vi "Recipe compare.vi"(8 "Recipe 2":T1={"SEM Scan Parameters"={"X size (um)"=20.0, "Y size (um)"=20.0, "X center (um)"=0.0, "Y center (um)"=0.0, "X size (V)"=6.190428211586902, "X size auto"=TRUE, "X stig"=[[0.0]], "Y stig"=[[0.0]], "X aln"=[[0.0]], "Y aln"=[[0.0]], "Scan rate (Hz)"=10000000, "Oversampling"=5, "Oversampling auto"=TRUE, "Frame line rampdown ratio"=0.1, "Pixel size (nm)"=10.0, "WD (mm)"=[[3.0]], "X tiles"=1, "Y tiles"=1, "Overlap (um)"=1.0, "Interlaced"=TRUE, "dX (um)"=0.0, "dY (um)"=0.0}, "Detector Information"={"Brightness A"=30.0, "Contrast A"=25.0, "Detector B name"="ESB", "Brightness B"=40.0, "Contrast B"=50.0, "Detector C name"="Detector C", "Detector D name"="Detector D"}, "SEM Options"={"GetInfo"=TRUE, "Set Det A para"=TRUE, "Set WD"=FALSE, "Set Mag"=TRUE, "Set stig"=FALSE, "Set aln"=FALSE, "Display"=TRUE, "Save"=TRUE, "Detector A"=TRUE, "Detector B"=FALSE, "Detector C"=FALSE, "Detector D"=FALSE, "Inverse A"=FALSE, "Inverse B"=FALSE, "Inverse C"=FALSE, "Inverse D"=FALSE, "Inverse PNG"=TRUE, "Freeze"=TRUE, "PNG only"=FALSE, "Upload"=TRUE, "Delete after upload"=FALSE}, "Keep aspect ratio"=TRUE, "Show Focus Index"=TRUE, "Focus Index primary grid center"=TRUE, "Focus Index grid X"=1, "Focus Index grid Y"=1, "Focus Index primary X grid"=0, "Focus Index primary Y grid"=0, "Image fit to"=0, "File Information"={"File path"=path "E:/Images", "Notes"="", "Save recipe"=FALSE, "Load recipe"=FALSE, "Sample ID"=""}, "Low mag SEM"={"Low mag scan"=TRUE, "Prior to main scan"=FALSE, "Low mag interval"=1, "Low mag scan FOV (micron)"=200.0, "Low mag scan rate (Hz)"=1000000, "Show HM box"=TRUE}, "Mid Mag SEM"={"Mid mag scan"=FALSE, "Prior to main scan"=FALSE, "Mid mag interval"=500, "X size (um)"=6144.0, "Y size (um)"=6144.0, "X center (um)"=0.0, "Y center (um)"=0.0, "Mid mag scan rate (Hz)"=1000000, "Pixel size (nm)"=10.0, "Show MM box"=TRUE}, "FIB-SEM Angle"=90.0, "Milling para"={"X resolution"=4096, "Y resolution"=100001, "X offset (um)"=0.0, "Y offset (um)"=0.0, "X center (um)"=0.0, "Y center (um)"=0.0, "X size (um)"=250.0, "Y size (um)"=250.0, "UL-Ang"=90.0, "UR-Ang"=90.0, "Line milling time (s)"=5.0, "Auto pause"=FALSE, "Lines auto pause"=1, "Mill from Bottom"=FALSE, "FIB FOV (um)"=500.0, "SEM on"=FALSE, "Mill start from Last"=FALSE, "FIB PID on"=FALSE, "FIB PID reset"=FALSE, "FIB PID measured"=0, "FIB PID target"=0.0, "FIB PID target slope"=0.0, "FIB PID P"=0.0, "FIB PID I"=0.0, "FIB PID D"=0.0}, "FI Detector"=0, "Auto Optimzation"=TRUE, "Images per Auto Optimization"=200, "AF Range (nm)"=1800.0, "AF Steps"=7, "AS Range (%)"=0.6, "AS Steps"=7, "AA Range (%)"=3.0, "AA Steps"=7, "X shift (nm/frame)"=0.0, "Y shift (nm/frame)"=0.0, "FIB Settings"={"Z-step (nm)"=2.5, "Enable alarm"=TRUE, "Label"="Emission Alarm (nA)", "Emission min"=1.2, "Emission max"=2.2, "Auto reheat"=FALSE}, "FIB Y zoom pixel (nm)"=20.0, "Mail server"="mail.hhmi.org", "Email Alert Recipents"=["xuc@janelia.hhmi.org"], "Alert Settings"={"3D imaging paused alarm"=TRUE, "FIB emission limit warning"=TRUE, "Low limit"=17.0, "High limit"=23.0, "Specimen current alarm "=TRUE, "Beam dump alarm"=TRUE, "EHT off alarm"=TRUE, "Temperature alarm"=TRUE, "Pause 3D-ING"=FALSE, "Low limit (F)"=70.0, "High limit (F)"=80.0, "Temp limit auto"=TRUE, "Delta (F)"=0.2, "Gradient limit (F/min)"=0.03, "SW error warning"=TRUE, "Focus index warning"=TRUE, "Focus index low limit"=0.1, "Focus index stop limit"=0.0, "Run Auto Stig"=FALSE, "FI low limit auto"=TRUE, "FI stop limit auto"=TRUE}, "Reheat Parameters"={"Filament I (A)"=3.0, "Reheat time (s)"=45.0, "Emission (uA)"=2.2, "Calculate V/I slope"=TRUE, "Pre-calc delay (min)"=5.0, "Disable Reheat Retries"=FALSE, "Restore Voltages"=TRUE}, "Start FIB HV DataLog"=FALSE, "Interval (s)"=60} {"SEM Scan Parameters"."dX (um)" step=1 format="%.2f"; "SEM Scan Parameters"."dY (um)" step=1 format="%.2f"; "SEM Scan Parameters"."WD (mm)" format="%.1f"; "SEM Scan Parameters"."Y aln" format="%.1f"; "SEM Scan Parameters"."X aln" format="%.1f"; "SEM Scan Parameters"."Y stig" format="%.1f"; "SEM Scan Parameters"."X stig" format="%.1f"; "SEM Scan Parameters"."Overlap (um)" min=0; "SEM Scan Parameters"."Y tiles" min=1; "SEM Scan Parameters"."X tiles" min=1; "SEM Scan Parameters"."X size (um)" format="%.2f"; "SEM Scan Parameters"."Y size (um)" format="%.2f"; "SEM Scan Parameters"."Frame line rampdown ratio" min=0 max=1 step=0.05 format="%.2g"; "SEM Scan Parameters"."X center (um)" step=1.0 format="%.2f"; "SEM Scan Parameters"."Y center (um)" step=1.0 format="%.2f"; "SEM Scan Parameters"."X size (V)" format="%_4g"; "SEM Scan Parameters"."Scan rate (Hz)" max=4000000 step=100000 format="%.2e"; "Reheat Parameters"."Pre-calc delay (min)" format="%.2f"; "Reheat Parameters"."Emission (uA)" format="%.1f"; "Reheat Parameters"."Filament I (A)" format="%.2f"; "Reheat Parameters"."Reheat time (s)" format="%.1f"; "Image fit to" items=["Width", "Height"]; "Mid Mag SEM"."X center (um)" step=1.0 format="%.4f"; "Mid Mag SEM"."Y center (um)" step=1.0 format="%.4f"; "Mid Mag SEM"."Mid mag interval" min=1 step=1; "Mid Mag SEM"."Mid mag scan rate (Hz)" max=4000000 step=100000 format="%.2e"; "Alert Settings"."Focus index stop limit" format="%_3g"; "Milling para"."FIB PID measured" items=["Spec.", "B.D."]; "Milling para"."UR-Ang" format="%.2f"; "Milling para"."UL-Ang" format="%.2f"; "Milling para"."Y offset (um)" step=0.02 format="%.3g"; "Milling para"."X offset (um)" step=1 format="%.3g"; "Milling para"."FIB FOV (um)" format="%.3g"; "Milling para"."Line milling time (s)" format="%.1f"; "Milling para"."Y center (um)" format="%#.3g"; "Milling para"."X center (um)" format="%#.3g"; "Focus Index grid X" min=1; "Focus Index grid Y" min=1; "FIB Y zoom pixel (nm)" format="%.1g"; "FIB Settings"."Emission min" format="%.1g"; "FIB Settings"."Emission max" format="%.1g"; "X shift (nm/frame)" step=0.1; "Y shift (nm/frame)" step=0.1; "FI Detector" items=["A", "B", "C", "D"]; "Low mag SEM"."Low mag interval" min=1 step=1; "Low mag SEM"."Low mag scan rate (Hz)" max=4000000 step=100000 format="%.2e"; "Low mag SEM"."Low mag scan FOV (micron)" step=50.0; "FIB-SEM Angle" min=0.0 max=90.0}, 11 "Recipe 1":T1={"SEM Scan Parameters"={"X size (um)"=20.0, "Y size (um)"=20.0, "X center (um)"=0.0, "Y center (um)"=0.0, "X size (V)"=6.190428211586902, "X size auto"=TRUE, "X stig"=[[0.0]], "Y stig"=[[0.0]], "X aln"=[[0.0]], "Y aln"=[[0.0]], "Scan rate (Hz)"=10000000, "Oversampling"=5, "Oversampling auto"=TRUE, "Frame line rampdown ratio"=0.1, "Pixel size (nm)"=10.0, "WD (mm)"=[[3.0]], "X tiles"=1, "Y tiles"=1, "Overlap (um)"=1.0, "Interlaced"=TRUE, "dX (um)"=0.0, "dY (um)"=0.0}, "Detector Information"={"Brightness A"=30.0, "Contrast A"=25.0, "Detector B name"="ESB", "Brightness B"=40.0, "Contrast B"=50.0, "Detector C name"="Detector C", "Detector D name"="Detector D"}, "SEM Options"={"GetInfo"=TRUE, "Set Det A para"=TRUE, "Set WD"=FALSE, "Set Mag"=TRUE, "Set stig"=FALSE, "Set aln"=FALSE, "Display"=TRUE, "Save"=TRUE, "Detector A"=TRUE, "Detector B"=FALSE, "Detector C"=FALSE, "Detector D"=FALSE, "Inverse A"=FALSE, "Inverse B"=FALSE, "Inverse C"=FALSE, "Inverse D"=FALSE, "Inverse PNG"=TRUE, "Freeze"=TRUE, "PNG only"=FALSE, "Upload"=TRUE, "Delete after upload"=FALSE}, "Keep aspect ratio"=TRUE, "Show Focus Index"=TRUE, "Focus Index primary grid center"=TRUE, "Focus Index grid X"=1, "Focus Index grid Y"=1, "Focus Index primary X grid"=0, "Focus Index primary Y grid"=0, "Image fit to"=0, "File Information"={"File path"=path "E:/Images", "Notes"="", "Save recipe"=FALSE, "Load recipe"=FALSE, "Sample ID"=""}, "Low mag SEM"={"Low mag scan"=TRUE, "Prior to main scan"=FALSE, "Low mag interval"=1, "Low mag scan FOV (micron)"=200.0, "Low mag scan rate (Hz)"=1000000, "Show HM box"=TRUE}, "Mid Mag SEM"={"Mid mag scan"=FALSE, "Prior to main scan"=FALSE, "Mid mag interval"=500, "X size (um)"=6144.0, "Y size (um)"=6144.0, "X center (um)"=0.0, "Y center (um)"=0.0, "Mid mag scan rate (Hz)"=1000000, "Pixel size (nm)"=10.0, "Show MM box"=TRUE}, "FIB-SEM Angle"=90.0, "Milling para"={"X resolution"=4096, "Y resolution"=100001, "X offset (um)"=0.0, "Y offset (um)"=0.0, "X center (um)"=0.0, "Y center (um)"=0.0, "X size (um)"=250.0, "Y size (um)"=250.0, "UL-Ang"=90.0, "UR-Ang"=90.0, "Line milling time (s)"=5.0, "Auto pause"=FALSE, "Lines auto pause"=1, "Mill from Bottom"=FALSE, "FIB FOV (um)"=500.0, "SEM on"=FALSE, "Mill start from Last"=FALSE, "FIB PID on"=FALSE, "FIB PID reset"=FALSE, "FIB PID measured"=0, "FIB PID target"=0.0, "FIB PID target slope"=0.0, "FIB PID P"=0.0, "FIB PID I"=0.0, "FIB PID D"=0.0}, "FI Detector"=0, "Auto Optimzation"=TRUE, "Images per Auto Optimization"=200, "AF Range (nm)"=1800.0, "AF Steps"=7, "AS Range (%)"=0.6, "AS Steps"=7, "AA Range (%)"=3.0, "AA Steps"=7, "X shift (nm/frame)"=0.0, "Y shift (nm/frame)"=0.0, "FIB Settings"={"Z-step (nm)"=2.5, "Enable alarm"=TRUE, "Label"="Emission Alarm (nA)", "Emission min"=1.2, "Emission max"=2.2, "Auto reheat"=FALSE}, "FIB Y zoom pixel (nm)"=20.0, "Mail server"="mail.hhmi.org", "Email Alert Recipents"=["xuc@janelia.hhmi.org"], "Alert Settings"={"3D imaging paused alarm"=TRUE, "FIB emission limit warning"=TRUE, "Low limit"=17.0, "High limit"=23.0, "Specimen current alarm "=TRUE, "Beam dump alarm"=TRUE, "EHT off alarm"=TRUE, "Temperature alarm"=TRUE, "Pause 3D-ING"=FALSE, "Low limit (F)"=70.0, "High limit (F)"=80.0, "Temp limit auto"=TRUE, "Delta (F)"=0.2, "Gradient limit (F/min)"=0.03, "SW error warning"=TRUE, "Focus index warning"=TRUE, "Focus index low limit"=0.1, "Focus index stop limit"=0.0, "Run Auto Stig"=FALSE, "FI low limit auto"=TRUE, "FI stop limit auto"=TRUE}, "Reheat Parameters"={"Filament I (A)"=3.0, "Reheat time (s)"=45.0, "Emission (uA)"=2.2, "Calculate V/I slope"=TRUE, "Pre-calc delay (min)"=5.0, "Disable Reheat Retries"=FALSE, "Restore Voltages"=TRUE}, "Start FIB HV DataLog"=FALSE, "Interval (s)"=60} {"SEM Scan Parameters"."dX (um)" step=1 format="%.2f"; "SEM Scan Parameters"."dY (um)" step=1 format="%.2f"; "SEM Scan Parameters"."WD (mm)" format="%.1f"; "SEM Scan Parameters"."Y aln" format="%.1f"; "SEM Scan Parameters"."X aln" format="%.1f"; "SEM Scan Parameters"."Y stig" format="%.1f"; "SEM Scan Parameters"."X stig" format="%.1f"; "SEM Scan Parameters"."Overlap (um)" min=0; "SEM Scan Parameters"."Y tiles" min=1; "SEM Scan Parameters"."X tiles" min=1; "SEM Scan Parameters"."X size (um)" format="%.2f"; "SEM Scan Parameters"."Y size (um)" format="%.2f"; "SEM Scan Parameters"."Frame line rampdown ratio" min=0 max=1 step=0.05 format="%.2g"; "SEM Scan Parameters"."X center (um)" step=1.0 format="%.2f"; "SEM Scan Parameters"."Y center (um)" step=1.0 format="%.2f"; "SEM Scan Parameters"."X size (V)" format="%_4g"; "SEM Scan Parameters"."Scan rate (Hz)" max=4000000 step=100000 format="%.2e"; "Reheat Parameters"."Pre-calc delay (min)" format="%.2f"; "Reheat Parameters"."Emission (uA)" format="%.1f"; "Reheat Parameters"."Filament I (A)" format="%.2f"; "Reheat Parameters"."Reheat time (s)" format="%.1f"; "Image fit to" items=["Width", "Height"]; "Mid Mag SEM"."X center (um)" step=1.0 format="%.4f"; "Mid Mag SEM"."Y center (um)" step=1.0 format="%.4f"; "Mid Mag SEM"."Mid mag interval" min=1 step=1; "Mid Mag SEM"."Mid mag scan rate (Hz)" max=4000000 step=100000 format="%.2e"; "Alert Settings"."Focus index stop limit" format="%_3g"; "Milling para"."FIB PID measured" items=["Spec.", "B.D."]; "Milling para"."UR-Ang" format="%.2f"; "Milling para"."UL-Ang" format="%.2f"; "Milling para"."Y offset (um)" step=0.02 format="%.3g"; "Milling para"."X offset (um)" step=1 format="%.3g"; "Milling para"."FIB FOV (um)" format="%.3g"; "Milling para"."Line milling time (s)" format="%.1f"; "Milling para"."Y center (um)" format="%#.3g"; "Milling para"."X center (um)" format="%#.3g"; "Focus Index grid X" min=1; "Focus Index grid Y" min=1; "FIB Y zoom pixel (nm)" format="%.1g"; "FIB Settings"."Emission min" format="%.1g"; "FIB Settings"."Emission max" format="%.1g"; "X shift (nm/frame)" step=0.1; "Y shift (nm/frame)" step=0.1; "FI Detector" items=["A", "B", "C", "D"]; "Low mag SEM"."Low mag interval" min=1 step=1; "Low mag SEM"."Low mag scan rate (Hz)" max=4000000 step=100000 format="%.2e"; "Low mag SEM"."Low mag scan FOV (micron)" step=50.0; "FIB-SEM Angle" min=0.0 max=90.0}) -> (3 "Recipe identical":bool)   [LabVIEW 2012]
panel:
  # "Images"
  # "nm"
  # "%"
  # "%"
  # "Direction"
  # "Start\nfrom"
  # "Det"
  # "after"
  # "Recipe"
  # "Brightness & Contrast (%)"
  # "Detector A"
  # "Brightness & Contrast (%)"
  # "Images"
  # "nm"
  # "%"
  # "%"
  # "Direction"
  # "Start\nfrom"
  # "Det"
  # "after"
  # "Recipe"
  # "Brightness & Contrast (%)"
  # "Detector A"
  # "Brightness & Contrast (%)"
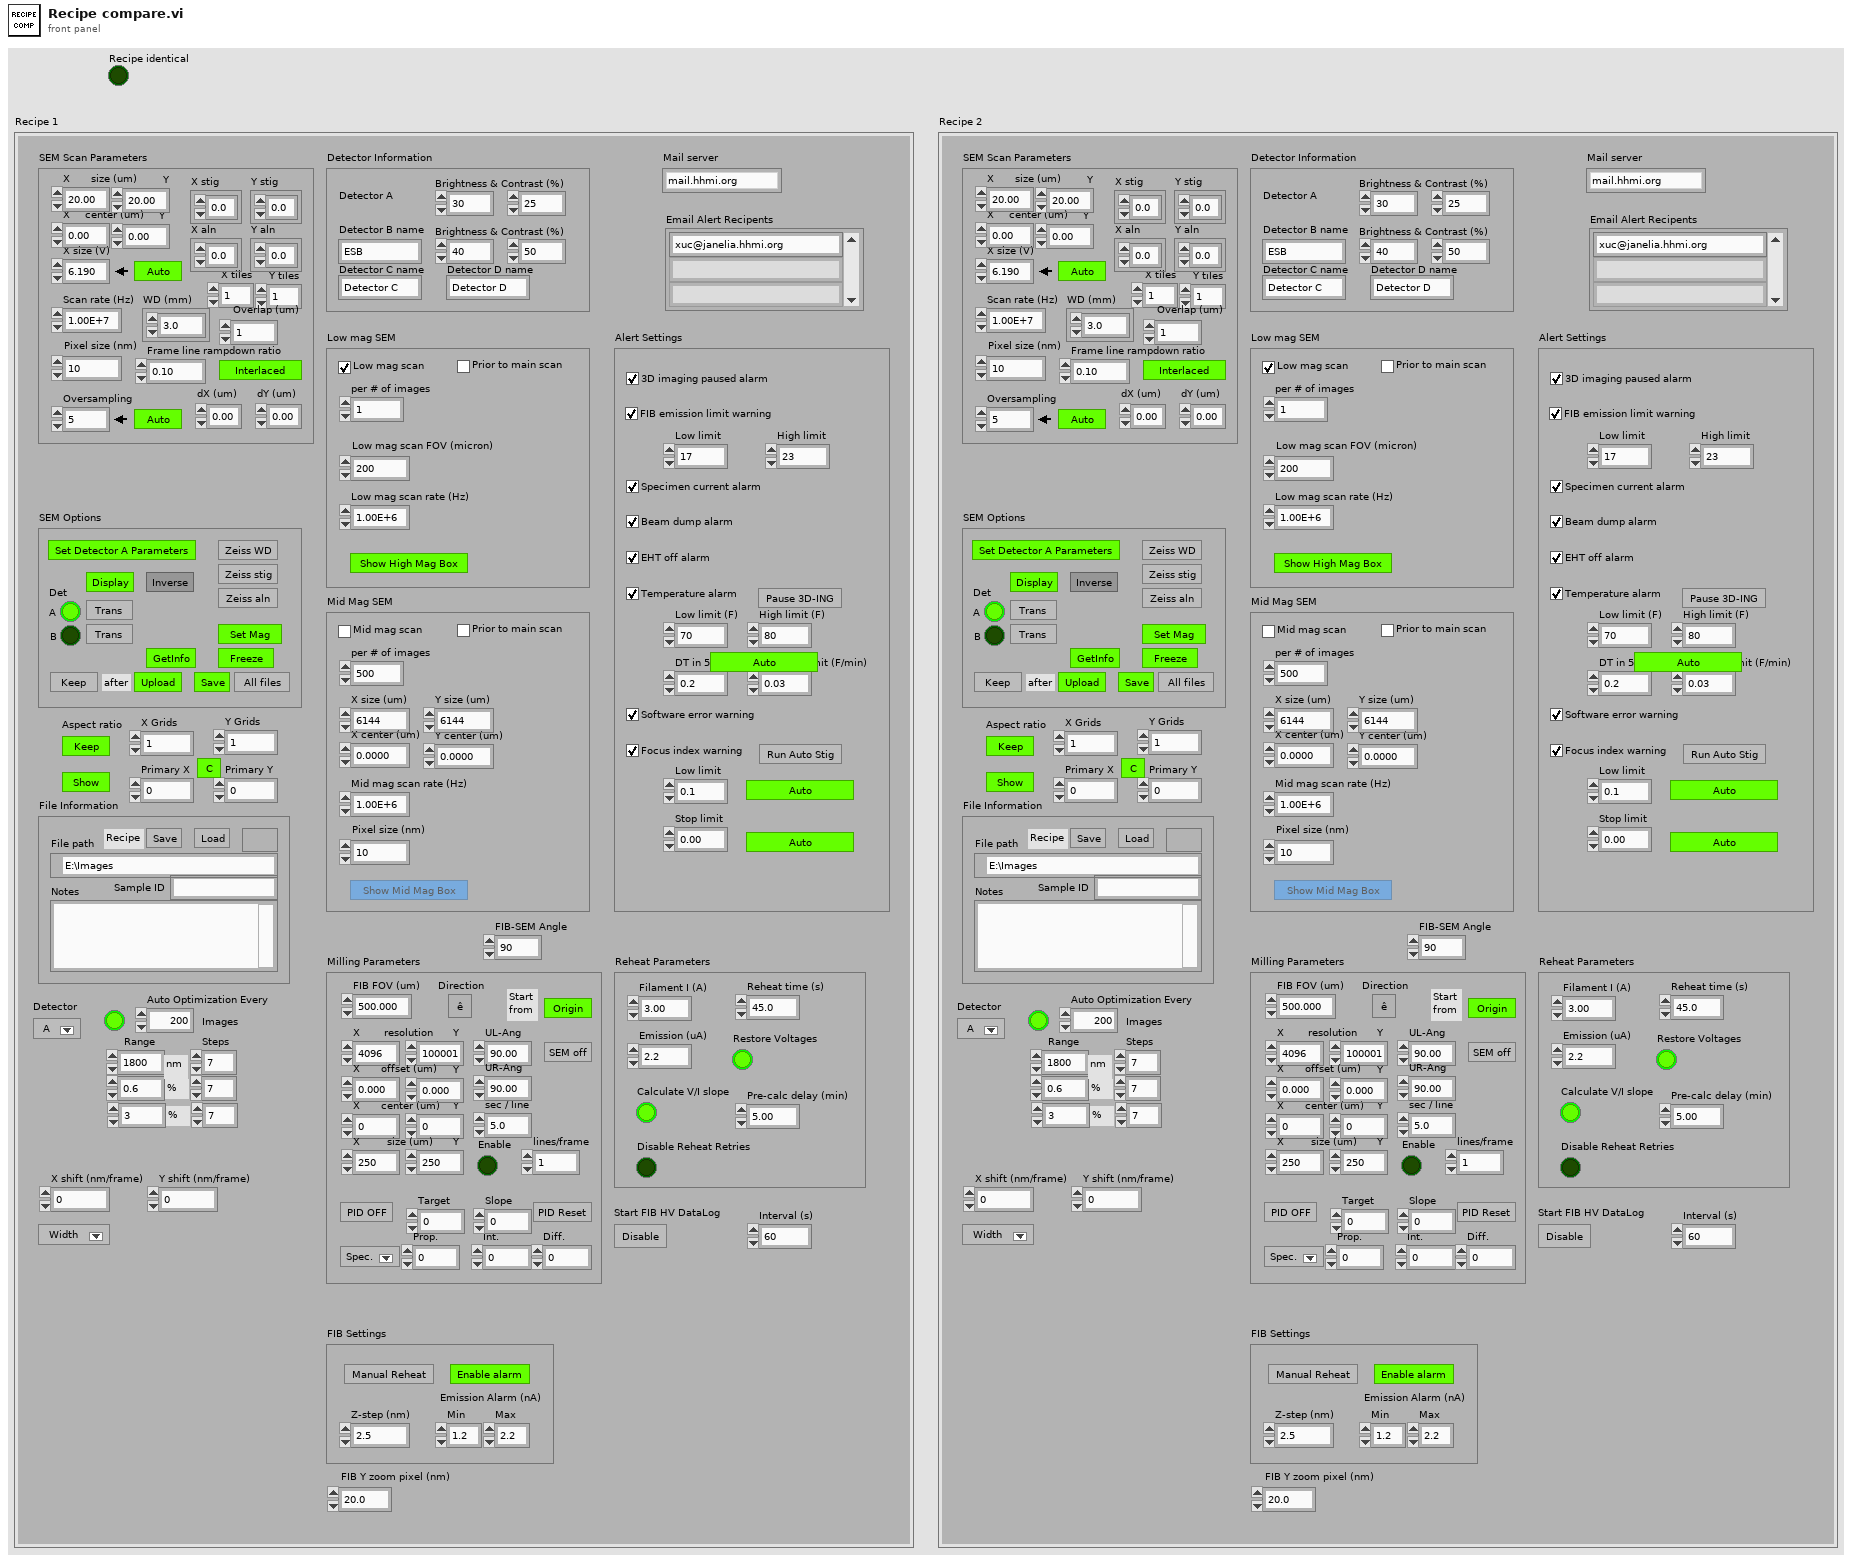
[diagram p1: front panel]
types:
  T1 = cluster{"SEM Scan Parameters":cluster{"X size (um)":sgl, "Y size (um)":sgl, "X center (um)":dbl, "Y center (um)":dbl, "X size (V)":dbl, "X size auto":bool, "X stig":sgl[][], "Y stig":sgl[][], "X aln":sgl[][], "Y aln":sgl[][], "Scan rate (Hz)":u32, "Oversampling":u32, "Oversampling auto":bool, "Frame line rampdown ratio":sgl, "Pixel size (nm)":sgl, "WD (mm)":sgl[][], "X tiles":u8, "Y tiles":u8, "Overlap (um)":sgl, "Interlaced":bool, "dX (um)":sgl, "dY (um)":sgl}, "Detector Information":cluster{"Brightness A":dbl, "Contrast A":dbl, "Detector B name":string, "Brightness B":dbl, "Contrast B":dbl, "Detector C name":string, "Detector D name":string}, "SEM Options":cluster{"GetInfo":bool, "Set Det A para":bool, "Set WD":bool, "Set Mag":bool, "Set stig":bool, "Set aln":bool, "Display":bool, "Save":bool, "Detector A":bool, "Detector B":bool, "Detector C":bool, "Detector D":bool, "Inverse A":bool, "Inverse B":bool, "Inverse C":bool, "Inverse D":bool, "Inverse PNG":bool, "Freeze":bool, "PNG only":bool, "Upload":bool, "Delete after upload":bool}, "Keep aspect ratio":bool, "Show Focus Index":bool, "Focus Index primary grid center":bool, "Focus Index grid X":u8, "Focus Index grid Y":u8, "Focus Index primary X grid":u8, "Focus Index primary Y grid":u8, "Image fit to":u8, "File Information":cluster{"File path":path, "Notes":string, "Save recipe":bool, "Load recipe":bool, "Sample ID":string}, "Low mag SEM":cluster{"Low mag scan":bool, "Prior to main scan":bool, "Low mag interval":u32, "Low mag scan FOV (micron)":dbl, "Low mag scan rate (Hz)":u32, "Show HM box":bool}, "Mid Mag SEM":cluster{"Mid mag scan":bool, "Prior to main scan":bool, "Mid mag interval":u32, "X size (um)":sgl, "Y size (um)":sgl, "X center (um)":dbl, "Y center (um)":dbl, "Mid mag scan rate (Hz)":u32, "Pixel size (nm)":dbl, "Show MM box":bool}, "FIB-SEM Angle":dbl, "Milling para":cluster{"X resolution":u32, "Y resolution":u32, "X offset (um)":sgl, "Y offset (um)":sgl, "X center (um)":sgl, "Y center (um)":sgl, "X size (um)":sgl, "Y size (um)":sgl, "UL-Ang":sgl, "UR-Ang":sgl, "Line milling time (s)":sgl, "Auto pause":bool, "Lines auto pause":u16, "Mill from Bottom":bool, "FIB FOV (um)":sgl, "SEM on":bool, "Mill start from Last":bool, "FIB PID on":bool, "FIB PID reset":bool, "FIB PID measured":u8, "FIB PID target":sgl, "FIB PID target slope":sgl, "FIB PID P":sgl, "FIB PID I":sgl, "FIB PID D":sgl}, "FI Detector":u16, "Auto Optimzation":bool, "Images per Auto Optimization":u16, "AF Range (nm)":dbl, "AF Steps":u8, "AS Range (%)":dbl, "AS Steps":u8, "AA Range (%)":sgl, "AA Steps":u8, "X shift (nm/frame)":dbl, "Y shift (nm/frame)":dbl, "FIB Settings":cluster{"Z-step (nm)":dbl, "Enable alarm":bool, "Label":string, "Emission min":dbl, "Emission max":dbl, "Auto reheat":bool}, "FIB Y zoom pixel (nm)":dbl, "Mail server":string, "Email Alert Recipents":string[], "Alert Settings":cluster{"3D imaging paused alarm":bool, "FIB emission limit warning":bool, "Low limit":dbl, "High limit":dbl, "Specimen current alarm ":bool, "Beam dump alarm":bool, "EHT off alarm":bool, "Temperature alarm":bool, "Pause 3D-ING":bool, "Low limit (F)":sgl, "High limit (F)":sgl, "Temp limit auto":bool, "Delta (F)":sgl, "Gradient limit (F/min)":sgl, "SW error warning":bool, "Focus index warning":bool, "Focus index low limit":dbl, "Focus index stop limit":sgl, "Run Auto Stig":bool, "FI low limit auto":bool, "FI stop limit auto":bool}, "Reheat Parameters":cluster{"Filament I (A)":sgl, "Reheat time (s)":sgl, "Emission (uA)":sgl, "Calculate V/I slope":bool, "Pre-calc delay (min)":sgl, "Disable Reheat Retries":bool, "Restore Voltages":bool}, "Start FIB HV DataLog":bool, "Interval (s)":u16}
  T2 = cluster{"SEM Scan Parameters":cluster{"X size (um)":bool, "Y size (um)":bool, "X center (um)":bool, "Y center (um)":bool, "X size (V)":bool, "X size auto":bool, "X stig":bool[][], "Y stig":bool[][], "X aln":bool[][], "Y aln":bool[][], "Scan rate (Hz)":bool, "Oversampling":bool, "Oversampling auto":bool, "Frame line rampdown ratio":bool, "Pixel size (nm)":bool, "WD (mm)":bool[][], "X tiles":bool, "Y tiles":bool, "Overlap (um)":bool, "Interlaced":bool, "dX (um)":bool, "dY (um)":bool}, "Detector Information":cluster{"Brightness A":bool, "Contrast A":bool, "Detector B name":bool, "Brightness B":bool, "Contrast B":bool, "Detector C name":bool, "Detector D name":bool}, "SEM Options":cluster{"GetInfo":bool, "Set Det A para":bool, "Set WD":bool, "Set Mag":bool, "Set stig":bool, "Set aln":bool, "Display":bool, "Save":bool, "Detector A":bool, "Detector B":bool, "Detector C":bool, "Detector D":bool, "Inverse A":bool, "Inverse B":bool, "Inverse C":bool, "Inverse D":bool, "Inverse PNG":bool, "Freeze":bool, "PNG only":bool, "Upload":bool, "Delete after upload":bool}, "Keep aspect ratio":bool, "Show Focus Index":bool, "Focus Index primary grid center":bool, "Focus Index grid X":bool, "Focus Index grid Y":bool, "Focus Index primary X grid":bool, "Focus Index primary Y grid":bool, "Image fit to":bool, "File Information":cluster{"File path":bool, "Notes":bool, "Save recipe":bool, "Load recipe":bool, "Sample ID":bool}, "Low mag SEM":cluster{"Low mag scan":bool, "Prior to main scan":bool, "Low mag interval":bool, "Low mag scan FOV (micron)":bool, "Low mag scan rate (Hz)":bool, "Show HM box":bool}, "Mid Mag SEM":cluster{"Mid mag scan":bool, "Prior to main scan":bool, "Mid mag interval":bool, "X size (um)":bool, "Y size (um)":bool, "X center (um)":bool, "Y center (um)":bool, "Mid mag scan rate (Hz)":bool, "Pixel size (nm)":bool, "Show MM box":bool}, "FIB-SEM Angle":bool, "Milling para":cluster{"X resolution":bool, "Y resolution":bool, "X offset (um)":bool, "Y offset (um)":bool, "X center (um)":bool, "Y center (um)":bool, "X size (um)":bool, "Y size (um)":bool, "UL-Ang":bool, "UR-Ang":bool, "Line milling time (s)":bool, "Auto pause":bool, "Lines auto pause":bool, "Mill from Bottom":bool, "FIB FOV (um)":bool, "SEM on":bool, "Mill start from Last":bool, "FIB PID on":bool, "FIB PID reset":bool, "FIB PID measured":bool, "FIB PID target":bool, "FIB PID target slope":bool, "FIB PID P":bool, "FIB PID I":bool, "FIB PID D":bool}, "FI Detector":bool, "Auto Optimzation":bool, "Images per Auto Optimization":bool, "AF Range (nm)":bool, "AF Steps":bool, "AS Range (%)":bool, "AS Steps":bool, "AA Range (%)":bool, "AA Steps":bool, "X shift (nm/frame)":bool, "Y shift (nm/frame)":bool, "FIB Settings":cluster{"Z-step (nm)":bool, "Enable alarm":bool, "Label":bool, "Emission min":bool, "Emission max":bool, "Auto reheat":bool}, "FIB Y zoom pixel (nm)":bool, "Mail server":bool, "Email Alert Recipents":bool[], "Alert Settings":cluster{"3D imaging paused alarm":bool, "FIB emission limit warning":bool, "Low limit":bool, "High limit":bool, "Specimen current alarm ":bool, "Beam dump alarm":bool, "EHT off alarm":bool, "Temperature alarm":bool, "Pause 3D-ING":bool, "Low limit (F)":bool, "High limit (F)":bool, "Temp limit auto":bool, "Delta (F)":bool, "Gradient limit (F/min)":bool, "SW error warning":bool, "Focus index warning":bool, "Focus index low limit":bool, "Focus index stop limit":bool, "Run Auto Stig":bool, "FI low limit auto":bool, "FI stop limit auto":bool}, "Reheat Parameters":cluster{"Filament I (A)":bool, "Reheat time (s)":bool, "Emission (uA)":bool, "Calculate V/I slope":bool, "Pre-calc delay (min)":bool, "Disable Reheat Retries":bool, "Restore Voltages":bool}, "Start FIB HV DataLog":bool, "Interval (s)":bool}
  T3 = cluster{"X size (um)":bool, "Y size (um)":bool, "X center (um)":bool, "Y center (um)":bool, "X size (V)":bool, "X size auto":bool, "X stig":bool[][], "Y stig":bool[][], "X aln":bool[][], "Y aln":bool[][], "Scan rate (Hz)":bool, "Oversampling":bool, "Oversampling auto":bool, "Frame line rampdown ratio":bool, "Pixel size (nm)":bool, "WD (mm)":bool[][], "X tiles":bool, "Y tiles":bool, "Overlap (um)":bool, "Interlaced":bool, "dX (um)":bool, "dY (um)":bool}
  T4 = cluster{"Brightness A":bool, "Contrast A":bool, "Detector B name":bool, "Brightness B":bool, "Contrast B":bool, "Detector C name":bool, "Detector D name":bool}
  T5 = cluster{"GetInfo":bool, "Set Det A para":bool, "Set WD":bool, "Set Mag":bool, "Set stig":bool, "Set aln":bool, "Display":bool, "Save":bool, "Detector A":bool, "Detector B":bool, "Detector C":bool, "Detector D":bool, "Inverse A":bool, "Inverse B":bool, "Inverse C":bool, "Inverse D":bool, "Inverse PNG":bool, "Freeze":bool, "PNG only":bool, "Upload":bool, "Delete after upload":bool}
  T6 = cluster{"File path":bool, "Notes":bool, "Save recipe":bool, "Load recipe":bool, "Sample ID":bool}
  T7 = cluster{"Low mag scan":bool, "Prior to main scan":bool, "Low mag interval":bool, "Low mag scan FOV (micron)":bool, "Low mag scan rate (Hz)":bool, "Show HM box":bool}
  T8 = cluster{"Mid mag scan":bool, "Prior to main scan":bool, "Mid mag interval":bool, "X size (um)":bool, "Y size (um)":bool, "X center (um)":bool, "Y center (um)":bool, "Mid mag scan rate (Hz)":bool, "Pixel size (nm)":bool, "Show MM box":bool}
  T9 = cluster{"X resolution":bool, "Y resolution":bool, "X offset (um)":bool, "Y offset (um)":bool, "X center (um)":bool, "Y center (um)":bool, "X size (um)":bool, "Y size (um)":bool, "UL-Ang":bool, "UR-Ang":bool, "Line milling time (s)":bool, "Auto pause":bool, "Lines auto pause":bool, "Mill from Bottom":bool, "FIB FOV (um)":bool, "SEM on":bool, "Mill start from Last":bool, "FIB PID on":bool, "FIB PID reset":bool, "FIB PID measured":bool, "FIB PID target":bool, "FIB PID target slope":bool, "FIB PID P":bool, "FIB PID I":bool, "FIB PID D":bool}
  T10 = cluster{"Z-step (nm)":bool, "Enable alarm":bool, "Label":bool, "Emission min":bool, "Emission max":bool, "Auto reheat":bool}
  T11 = cluster{"3D imaging paused alarm":bool, "FIB emission limit warning":bool, "Low limit":bool, "High limit":bool, "Specimen current alarm ":bool, "Beam dump alarm":bool, "EHT off alarm":bool, "Temperature alarm":bool, "Pause 3D-ING":bool, "Low limit (F)":bool, "High limit (F)":bool, "Temp limit auto":bool, "Delta (F)":bool, "Gradient limit (F/min)":bool, "SW error warning":bool, "Focus index warning":bool, "Focus index low limit":bool, "Focus index stop limit":bool, "Run Auto Stig":bool, "FI low limit auto":bool, "FI stop limit auto":bool}
  T12 = cluster{"Filament I (A)":bool, "Reheat time (s)":bool, "Emission (uA)":bool, "Calculate V/I slope":bool, "Pre-calc delay (min)":bool, "Disable Reheat Retries":bool, "Restore Voltages":bool}
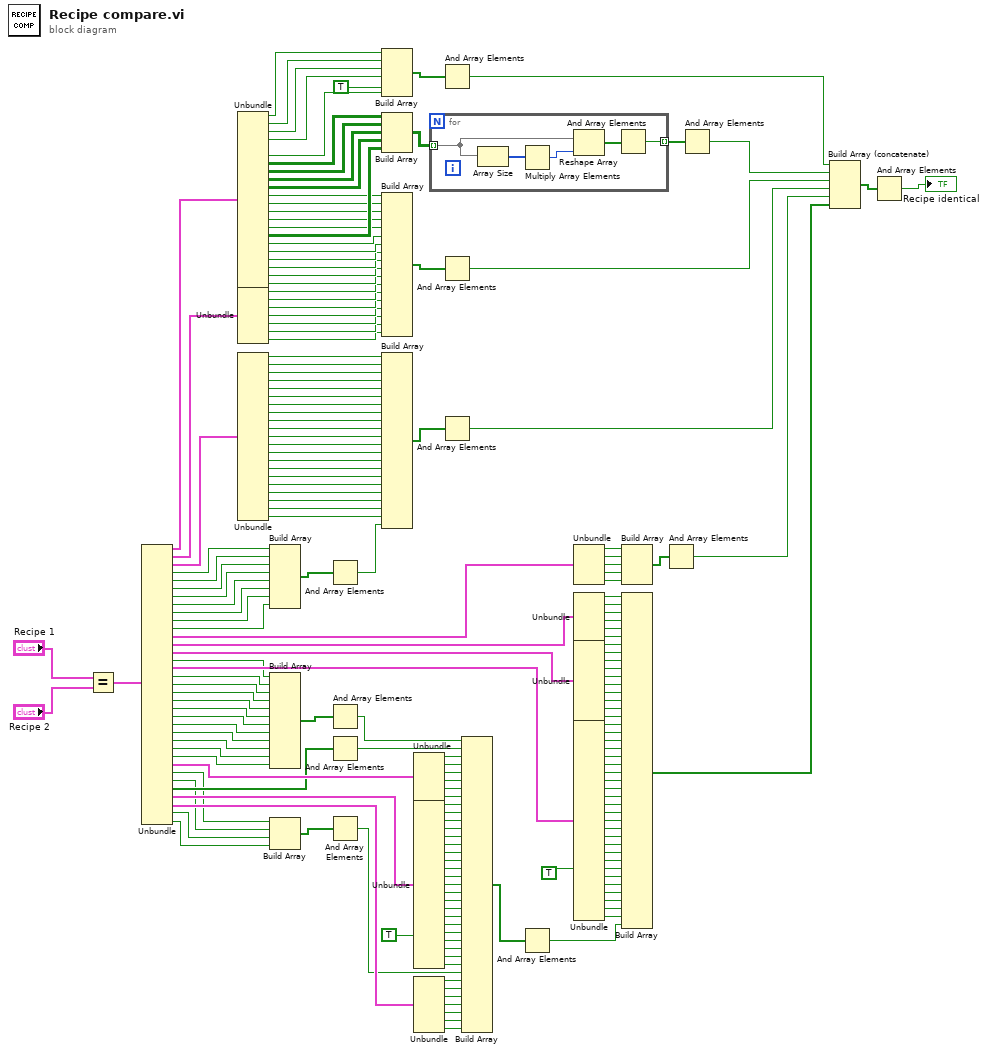
[diagram p0: block diagram]
diagram:
  n1 = Equal?(x="Recipe 1", y="Recipe 2") -> (x = y?=w181:T2)
  n2 = Unbundle(w181) -> ("SEM Scan Parameters"=w189:T3, "Detector Information"=w188:T4, "SEM Options"=w187:T5, "Keep aspect ratio"=w129:bool, "Show Focus Index"=w128:bool, "Focus Index primary grid center"=w127:bool, "Focus Index grid X"=w126:bool, "Focus Index grid Y"=w125:bool, "Focus Index primary X grid"=w124:bool, "Focus Index primary Y grid"=w123:bool, "Image fit to"=w122:bool, "File Information"=w132:T6, "Low mag SEM"=w131:T7, "Mid Mag SEM"=w130:T8, "FIB-SEM Angle"=w115:bool, "Milling para"=w119:T9, "FI Detector"=w114:bool, "Auto Optimzation"=w113:bool, "Images per Auto Optimization"=w112:bool, "AF Range (nm)"=w111:bool, "AF Steps"=w110:bool, "AS Range (%)"=w109:bool, "AS Steps"=w108:bool, "AA Range (%)"=w107:bool, "AA Steps"=w106:bool, "X shift (nm/frame)"=w105:bool, "Y shift (nm/frame)"=w104:bool, "FIB Settings"=w118:T10, "FIB Y zoom pixel (nm)"=w102:bool, "Mail server"=w100:bool, "Email Alert Recipents"=w103:bool[], "Alert Settings"=w117:T11, "Reheat Parameters"=w116:T12, "Start FIB HV DataLog"=w99:bool, "Interval (s)"=w98:bool)
  n3 = Unbundle(w189) -> ("X size (um)"=w186:bool, "Y size (um)"=w185:bool, "X center (um)"=w184:bool, "Y center (um)"=w183:bool, "X size auto"=w182:bool, "X stig"=w180:bool[][], "Y stig"=w179:bool[][], "X aln"=w178:bool[][], "Y aln"=w177:bool[][], "Scan rate (Hz)"=w172:bool, "Oversampling"=w171:bool, "Oversampling auto"=w170:bool, "Frame line rampdown ratio"=w169:bool, "Pixel size (nm)"=w168:bool, "WD (mm)"=w173:bool[][], "X tiles"=w167:bool, "Y tiles"=w166:bool, "Overlap (um)"=w165:bool, "Interlaced"=w164:bool, "dX (um)"=w163:bool, "dY (um)"=w162:bool)  [unwired: 1 out]
  n4 = Unbundle(w188) -> ("Brightness A"=w161:bool, "Contrast A"=w160:bool, "Detector B name"=w159:bool, "Brightness B"=w158:bool, "Contrast B"=w157:bool, "Detector C name"=w156:bool, "Detector D name"=w155:bool)
  n5 = Unbundle(w187) -> ("GetInfo"=w153:bool, "Set Det A para"=w152:bool, "Set WD"=w151:bool, "Set Mag"=w150:bool, "Set stig"=w149:bool, "Set aln"=w148:bool, "Display"=w147:bool, "Save"=w146:bool, "Detector A"=w145:bool, "Detector B"=w144:bool, "Detector C"=w143:bool, "Detector D"=w142:bool, "Inverse A"=w141:bool, "Inverse B"=w140:bool, "Inverse C"=w139:bool, "Inverse D"=w138:bool, "Inverse PNG"=w137:bool, "Freeze"=w136:bool, "PNG only"=w135:bool, "Upload"=w134:bool, "Delete after upload"=w133:bool)
  n6 = Build Array(w129, w128, w127, w126, w125, w124, w123, w122) -> (w120:bool[])
  n7 = Build Array(w115, w114, w113, w112, w111, w110, w109, w108, w107, w106, w105, w104) -> (w101:bool[])
  n8 = Build Array(w102, w100, w99, w98) -> (w97:bool[])
  n9 = And Array Elements(Boolean array=w120) -> (logical AND=w61:bool)
  n10 = And Array Elements(Boolean array=w101) -> (logical AND=w96:bool)
  n11 = And Array Elements(Boolean array=w103) -> (logical AND=w95:bool)
  n12 = And Array Elements(Boolean array=w97) -> (logical AND=w69:bool)
  n13 = Build Array(w186, w185, w184, w183, TRUE ("X size (um)"), w182) -> (w174:bool[])
  n14 = Build Array(w180, w179, w178, w177, w173) -> (w176:bool[][][])
  n15 = Build Array(w172, w171, w170, w169, w168, w167, w166, w165, w164, w163, w162, w161, w160, w159, w158, w157, w156, w155) -> (w154:bool[])
  n16 = Build Array(w153, w152, w151, w150, w149, w148, w147, w146, w145, w144, w143, w142, w141, w140, w139, w138, w137, w136, w135, w134, w133, w61) -> (w121:bool[])
  n17 = Unbundle(w118) -> ("Z-step (nm)"=w94:bool, "Enable alarm"=w93:bool, "Label"=w92:bool, "Emission min"=w91:bool, "Emission max"=w90:bool, "Auto reheat"=w89:bool)
  n18 = Unbundle(w117) -> ("3D imaging paused alarm"=w88:bool, "FIB emission limit warning"=w87:bool, "Low limit"=w86:bool, "High limit"=w85:bool, "Specimen current alarm"=w84:bool, "Beam dump alarm"=w83:bool, "EHT off alarm"=w82:bool, "Temperature alarm"=w81:bool, "Pause 3D-ING"=w80:bool, "Low limit (F)"=w79:bool, "High limit (F)"=w78:bool, "Temp limit auto"=w77:bool, "Delta (F)"=w76:bool, "Gradient limit (F/min)"=w75:bool, "SW error warning"=w74:bool, "Focus index warning"=w73:bool, "Focus index stop limit"=w3:bool, "Run Auto Stig"=w72:bool, "FI low limit auto"=w71:bool, "FI stop limit auto"=w70:bool)  [unwired: 1 out]
  n19 = Unbundle(w116) -> ("Filament I (A)"=w68:bool, "Reheat time (s)"=w67:bool, "Emission (uA)"=w66:bool, "Calculate V/I slope"=w65:bool, "Pre-calc delay (min)"=w64:bool, "Disable Reheat Retries"=w63:bool, "Restore Voltages"=w62:bool)
  n20 = for {
    tunnel: w176 -> [w194] mode=indexing
    tunnel: [w192] -> w175 mode=indexing
    n21 = Array Size(array=w194) -> (size(s)=w195:i32[])
    n22 = Multiply Array Elements(1:w195) -> (0:w196:i32)
    n23 = Reshape Array(w194, w196) -> (w193:bool[])
    n24 = And Array Elements(Boolean array=w193) -> (logical AND=w192:bool)
  }
  n25 = And Array Elements(Boolean array=w174) -> (logical AND=w13:bool)
  n26 = And Array Elements(Boolean array=w154) -> (logical AND=w11:bool)
  n27 = And Array Elements(Boolean array=w121) -> (logical AND=w10:bool)
  n28 = Build Array(w96, w95, w94, w93, w92, w91, w90, w89, w88, w87, w86, w85, w84, w83, w82, w81, w80, w79, w78, w77, w76, w75, w74, w73, TRUE ("element"), w3, w72, w71, w70, w69, w68, w67, w66, w65, w64, w63, w62) -> (w14:bool[])
  n29 = And Array Elements(Boolean array=w14) -> (logical AND=w7:bool)
  n30 = Unbundle(w132) -> ("File path"=w60:bool, "Notes"=w59:bool, "Save recipe"=w58:bool, "Load recipe"=w57:bool, "Sample ID"=w56:bool)
  n31 = Unbundle(w131) -> ("Low mag scan"=w54:bool, "Prior to main scan"=w53:bool, "Low mag interval"=w52:bool, "Low mag scan FOV (micron)"=w51:bool, "Low mag scan rate (Hz)"=w50:bool, "Show HM box"=w49:bool)
  n32 = Unbundle(w130) -> ("Mid mag scan"=w48:bool, "Prior to main scan"=w47:bool, "Mid mag interval"=w46:bool, "X size (um)"=w45:bool, "Y size (um)"=w44:bool, "X center (um)"=w42:bool, "Y center (um)"=w43:bool, "Mid mag scan rate (Hz)"=w41:bool, "Pixel size (nm)"=w40:bool, "Show MM box"=w39:bool)
  n33 = Unbundle(w119) -> ("X resolution"=w38:bool, "Y resolution"=w37:bool, "X offset (um)"=w36:bool, "Y offset (um)"=w35:bool, "X center (um)"=w34:bool, "Y center (um)"=w33:bool, "X size (um)"=w32:bool, "Y size (um)"=w31:bool, "UL-Ang"=w30:bool, "UR-Ang"=w29:bool, "Line milling time (s)"=w28:bool, "Auto pause"=w27:bool, "Lines auto pause"=w26:bool, "Mill from Bottom"=w25:bool, "FIB FOV (um)"=w24:bool, "SEM on"=w23:bool, "Mill start from Last"=w22:bool, "FIB PID on"=w21:bool, "FIB PID measured"=w20:bool, "FIB PID target"=w19:bool, "FIB PID target slope"=w18:bool, "FIB PID P"=w17:bool, "FIB PID I"=w16:bool, "FIB PID D"=w15:bool)  [unwired: 1 out]
  n34 = Build Array(w60, w59, w58, w57, w56) -> (w55:bool[])
  n35 = Build Array(w54, w53, w52, w51, w50, w49, w48, w47, w46, w45, w44, w42, w43, w41, w40, w39, w38, w37, w36, w35, w34, w33, w32, w31, w30, w29, w28, w27, w26, w25, w24, w23, w22, w21, TRUE ("element"), w20, w19, w18, w17, w16, w15, w7) -> (w8:bool[])
  n36 = And Array Elements(Boolean array=w55) -> (logical AND=w9:bool)
  n37 = And Array Elements(Boolean array=w175) -> (logical AND=w12:bool)
  n38 = Build Array (concatenate)(w13, w12, w11, w10, w9, w8) -> (w6:bool[])
  n39 = And Array Elements(Boolean array=w6) -> (logical AND=→"Recipe identical":bool)
